vi "LVClass_WavefrontCorrectorSet Save UsersPreferencesValue.vi"(0 "WavefrontCorrectorSet in":refnum<class "WavefrontCorrectorSet.lvclass">, 11 "error in (no error)":errorcluster) -> (4 "WavefrontCorrectorSet out":refnum<class "WavefrontCorrectorSet.lvclass">, 15 "error out":errorcluster)   [LabVIEW 2020, in "WavefrontCorrectorSet.lvclass"]
uses:
  WavefrontCorrectorSet.lvclass
  WavefrontCorrectorSet.lvclass/WavefrontCorrectorSet.ctl
  <vilib>/Utility/xml.llb/Write to XML File(string).vi
panel:
  in  "PreferencesValue file path":path
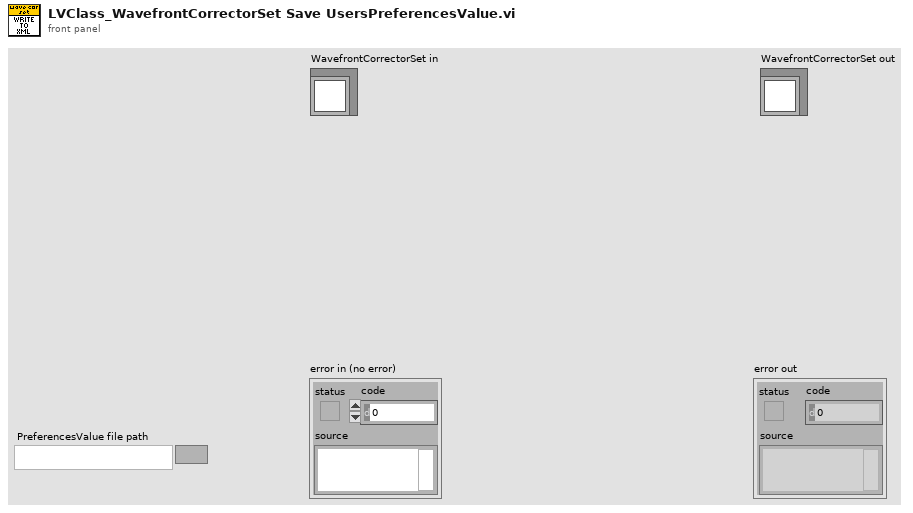
[diagram p1: front panel]
types:
  T1 = typedef "Wavefront Corrector states.ctl" = cluster{"Sleep after command apply_ms":i32, "Wavefront Corrector State":T2[], "WavefrontCorrectorOffsetState":sgl[]}
  T2 = typedef "Wavefront Corrector states - ONE.ctl" = cluster{"Max":sgl, "Min":sgl, "Validity":enum16{"valid", "fixed", "invalid"}, "Fixed_Position":sgl}
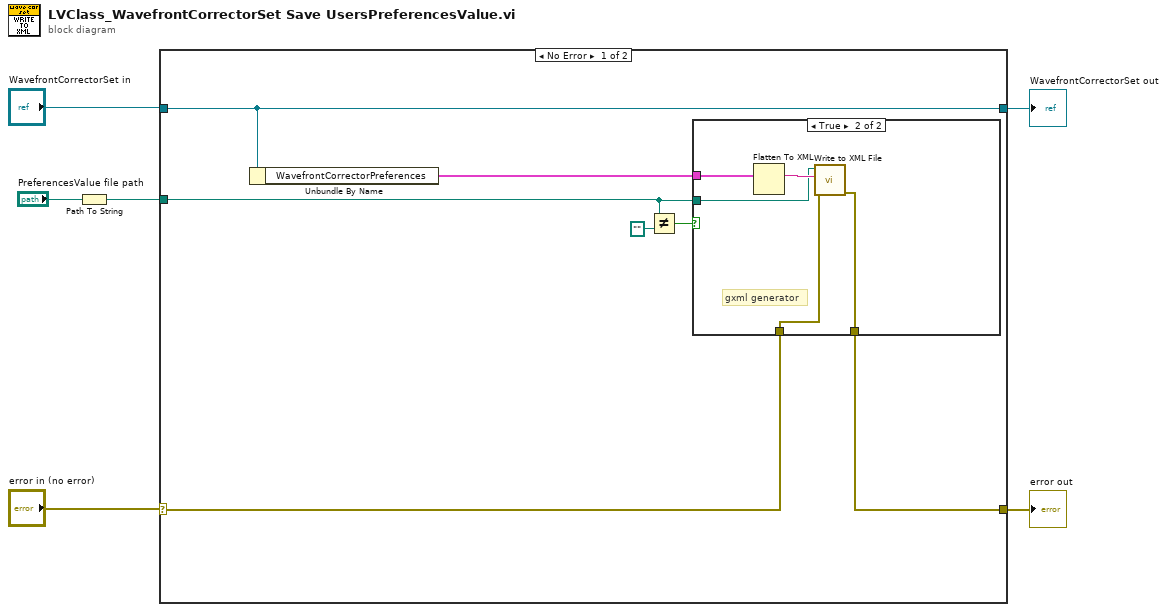
[diagram p0: block diagram]
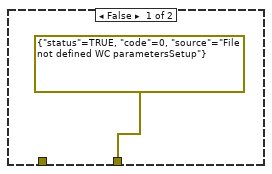
[diagram p2: hidden frame]
diagram:
  n1 = Path To String(path="PreferencesValue file path") -> ()  [unwired: 1 out]
  n2 = case shown="No Error" "error in (no error)" {
    selector: "error in (no error)" -> [w12 w20]
    tunnel: [w11 w20] -> w4
    tunnel: [w8 w19] -> w2
    tunnel: "WavefrontCorrectorSet in" -> [w8 w19]
    tunnel: "PreferencesValue file path" -> [w6 _]
    frame No Error {
      n3 = Unbundle By Name(w8) -> ("WavefrontCorrectorPreferences"=w7:T1)
      n4 = Not Equal?(x=w6, y=path "") -> (x != y?=w9:bool)
      n5 = case shown="True" w9 {
        tunnel: w7 -> [_ w17]
        tunnel: w6 -> [_ w16]
        tunnel: w12 -> [_ w14]
        tunnel: [errorcluster {"status"=TRUE, "code"=0, "source"="File not defined WC parametersSetup"} ("error out") w15] -> w11
        frame False {
        }
        frame True {
          # "gxml generator"
          n6 = Flatten To XML(6:w17) -> (2:w18:string)
          n7 = call-poly <vilib>:"Write to XML File.vi"("error in (no error)"=w14, "XML Input"=w18, "XML File Path"=w16) -> ("error out"=w15:errorcluster)  [unwired: 6 in, 2 out]
        }
      }
    }
    frame Error {
    }
  }
  "error out" <- w4
  "WavefrontCorrectorSet out" <- w2
